vi "Etalonnage.vi"(6 "GraphIn":cluster{dbl[], dbl[]}, 7 "Reference Cell":i32=1, 8 "error in":errorcluster, 9 "Sleeve":u32, 10 "Over":bool=TRUE, 11 "NextStep":bool=TRUE) -> (0 "error out":errorcluster, 1 "Résidu":dbl, 2 "CoeffsPoly":dbl[](array[numeric]), 3 "Values":cluster{dbl[], dbl[]})   [LabVIEW 2012]
uses:
  GlobalVariables/CalibrationVolumes.vi
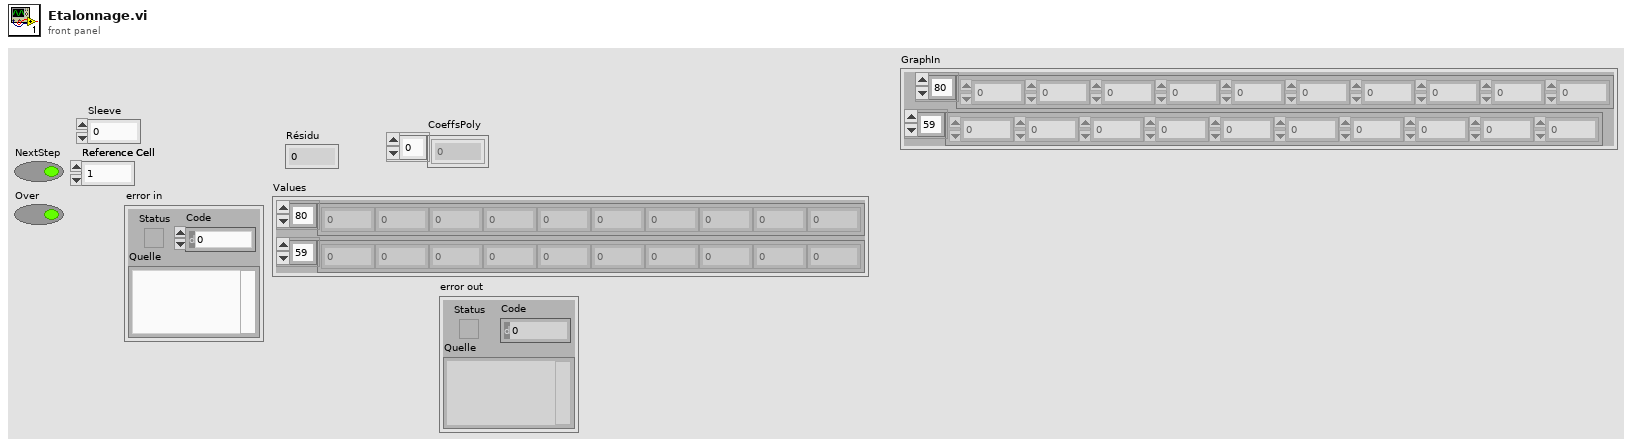
[diagram p1: front panel]
types:
  T1 = cluster{"CalibrationVolumes":dbl[], "SetName":string}[]
  T2 = cluster{"CalibrationVolumes":dbl[], "SetName":string}
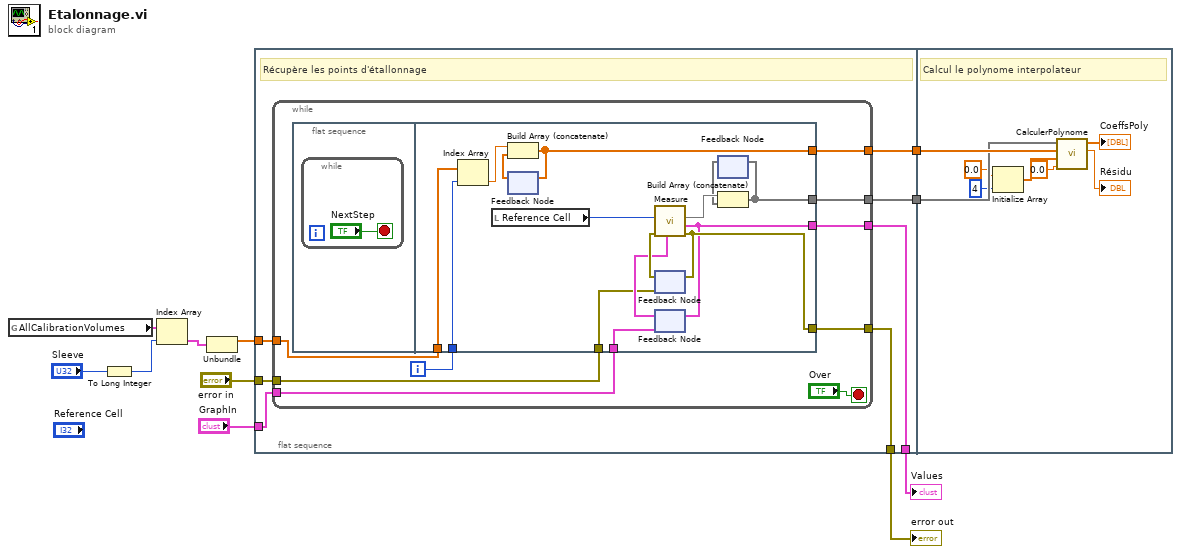
[diagram p0: block diagram]
diagram:
  n1 = global read "CalibrationVolumes.vi" "AllCalibrationVolumes"() -> (w7:T1)
  n2 = To Long Integer(number="Sleeve") -> (32bit integer=w2:i32)
  n3 = Index Array(array=w7, index=w2) -> (element=w6:T2)
  n4 = Unbundle(w6) -> ("CalibrationVolumes"=w5:dbl[])  [unwired: 1 out]
  n5 = flat-sequence {
    tunnel: [w18] -> w11
    tunnel: [w17] -> w10
    tunnel: [w16] -> w9
    tunnel: [w15] -> w8
    tunnel: w5 -> [w14]
    tunnel: "GraphIn" -> [w13]
    tunnel: "error in" -> [w12]
    tunnel: w11 -> [w51]
    tunnel: w10 -> [w50]
    frame #0 {
      # "Récupère les points d'étallonnage"
      n6 = while {
        tunnel: [w26] -> w15
        tunnel: [w25] -> w18
        tunnel: [w24] -> w17
        tunnel: [w23] -> w16
        tunnel: w14 -> [w21]
        tunnel: w13 -> [w20]
        tunnel: w12 -> [w19]
        i -> [w22]
        stop <- "Over" stop-if-true
        n7 = flat-sequence {
          tunnel: [w38] -> w26
          tunnel: [w37] -> w25
          tunnel: [w36] -> w24
          tunnel: [w35] -> w23
          tunnel: w22 -> [w33]
          tunnel: w21 -> [w31]
          tunnel: w20 -> [w30]
          tunnel: w19 -> [w29]
          frame #0 {
            n8 = while {
              stop <- "NextStep" stop-if-true
            }
          }
          frame #1 {
            n9 = Index Array(array=w31, index=w33) -> (element=w34:dbl)
            n10 = local read "Reference Cell"() -> (w32:i32)
            n11 = feedback #1() -> (w39:dbl[])  [unwired: 1 in]
            n12 = Build Array (concatenate)(w34, w39) -> (w37:dbl[])
            n13 = feedback-in #1(w37) -> ()
            n14 = feedback #2(w29) -> (w43:errorcluster)
            n15 = feedback #3(w30) -> (w42:cluster{dbl[], dbl[]})
            n16 = call "Measure.vi"("Graph in"=w42, "error in"=w43, 10:w32) -> ("error out"=w38:errorcluster, "Values"=w35:cluster{dbl[], dbl[]}, 2:w41)  [unwired: 5 in, 1 out]
            n17 = feedback-in #2(w38) -> ()
            n18 = feedback-in #3(w35) -> ()
            n19 = feedback #4() -> (w40:void[])  [unwired: 1 in]
            n20 = Build Array (concatenate)(w41, w40) -> (w36:void[])
            n21 = feedback-in #4(w36) -> ()
          }
        }
      }
    }
    frame #1 {
      # "Calcul le polynome interpolateur"
      n22 = Initialize Array(0.0, 4) -> (w47:dbl[])
      n23 = call "CalculerPolynome.vi"("e3 [in]"=0.0, "Meilleure poly [in]"=w47, "Y"=w51, "X"=w50) -> ("Résidu [out]"=→"Résidu":dbl, "Meilleur poly [out]"=→"CoeffsPoly":dbl[])  [unwired: 6 in]
    }
  }
  "Values" <- w9
  "error out" <- w8
